vi "Untitled 2.vi"() -> ()   [LabVIEW 2017]
uses:
  <vilib>/myRIO/Common/Instrument Driver Framework/myRIO v1.0/Encoder/typedefs/Encoder Signal Mode.ctl
  <vilib>/myRIO/Instrument Drivers/Onboard IO/Encoder/typedefs/Encoder Reference.ctl
  <vilib>/myRIO/Common/Instrument Driver Framework/Utilities/typedefs/myRIO Generic Hardware Reference.ctl
  <vilib>/myRIO/Common/Instrument Driver Framework/Utilities/typedefs/Hardware Version Enum.ctl
  <vilib>/myRIO/Common/Instrument Driver Framework/Utilities/typedefs/myRIO v1.0 Reference.ctl
  <vilib>/myRIO/Common/Instrument Driver Framework/Utilities/typedefs/Generic FPGA Reference.ctl
  <vilib>/myRIO/Common/Instrument Driver Framework/myRIO v1.0/Encoder/typedefs/Encoder Channels Enum.ctl
  <vilib>/myRIO/Common/Instrument Driver Framework/myRIO v1.0/Encoder/typedefs/Encoder Configuration v1.0.ctl
  <vilib>/userdefined/High Color/nirio_resource_hc.ctl
  <vilib>/myRIO/Common/Instrument Driver Framework/Utilities/vis/Is FPGA Ref Available.vi
  <vilib>/myRIO/Common/Instrument Driver Framework/myRIO v1.0/Encoder/vis/myRIO v1.1 Open Encoder.vi
  <vilib>/myRIO/Instrument Drivers/Onboard IO/Encoder/vis/Read.vi
  <vilib>/myRIO/Common/Instrument Driver Framework/Utilities/vis/Validate Channels.vi
  <vilib>/myRIO/Common/Instrument Driver Framework/myRIO v1.0/Encoder/vis/myRIO v1.0 Reserve Encoder.vi
  <vilib>/myRIO/Common/Instrument Driver Framework/myRIO v1.0/Encoder/vis/myRIO v1.0 Build MUX Configuration Encoder.vi
  <vilib>/myRIO/Common/Instrument Driver Framework/myRIO v1.0/Resource Manager/vis/myRIO v1.0 Reserve Channel List.vi
  <vilib>/myRIO/Common/Instrument Driver Framework/myRIO v1.0/Resource Manager/vis/myRIO v1.0 Create Configuration List.vi
  <vilib>/myRIO/Common/Instrument Driver Framework/myRIO v1.0/Resource Manager/vis/myRIO v1.0 Reserve Channel.vi
  <vilib>/myRIO/Common/Instrument Driver Framework/myRIO v1.0/Resource Manager/vis/myRIO v1.0 Unreserve Channel.vi
  <vilib>/myRIO/Common/Instrument Driver Framework/myRIO v1.0/Resource Manager/vis/myRIO v1.0 Build Mutex Name.vi
  <vilib>/Utility/VariantDataType/GetNumericInfo.vi
  <vilib>/Utility/error.llb/Error Cluster From Error Code.vi
  <vilib>/myRIO/Common/Instrument Driver Framework/myRIO v1.0/myRIO v1.1 Open.vi
  <vilib>/myRIO/Common/Instrument Driver Framework/Utilities/vis/IO Manager.vi
  <vilib>/myRIO/Common/Instrument Driver Framework/Utilities/vis/Configuration Manager.vi
  <vilib>/myRIO/Common/Instrument Driver Framework/myRIO v1.0/Resource Manager/vis/myRIO v1.0 Configure IO.vi
  <vilib>/myRIO/Common/Instrument Driver Framework/myRIO v1.0/myRIO v1.0 Close.vi
  <vilib>/myRIO/Common/Instrument Driver Framework/myRIO v1.0/Encoder/vis/myRIO v1.0 Configure Encoder.vi
  <vilib>/myRIO/Common/Instrument Driver Framework/myRIO v1.0/Encoder/vis/myRIO v1.0 Read Encoder.vi
  <vilib>/addons/control/pid/pid.llb/PID (DBL).vi
  <vilib>/myRIO/Express VI/Onboard IO/Encoder/Encoder Express VI.xnode
  <vilib>/myRIO/Instrument Drivers/Onboard IO/Encoder/vis/myRIO Encoder Open.xnode
  <vilib>/myRIO/Common/Instrument Driver Framework/myRIO v1.0/Encoder/typedefs/Encoder Count Direction Enum.ctl
  <vilib>/addons/control/pid/NI_PID_pid.lvlib
  <vilib>/myRIO/Instrument Drivers/Onboard IO/Encoder/Encoder.lvlib
  <vilib>/Analysis/NI_AALPro.lvlib
  <vilib>/robotics/Navigation/shared/WorldMap/OccupancyGridWorldMap/NI_Robotics_OccupancyGridWorldMap.lvclass
panel:
  out "XY Graph 2":cluster{dbl[], dbl[]}(graph)
  in  "stop 2":bool
  in  "Resolution":dbl=50.0
  out "Intensity Graph":dbl[][](graph)
  out "Frequency":u32=10
  in  "curPos":cluster{"x":i32, "y":i32}
  in  "endPos":cluster{"x":i32, "y":i32}={"x"=0, "y"=6}
  out "path":cluster{"X":i32, "Y":i32}[](array[cluster])
  out "Setpoint B":dbl(slide)=1.3993520911950799 scale=-10.0..10.0
  out "Setpoint A":dbl(slide)=0.6006479088049201 scale=-10.0..10.0
  out "PID B":T1(graph)={"Setpoint"=1.3993520911950799, "output"=0.10115092019020398, "dx/dt"=1.4}
  out "PID A":T1(graph)={"Setpoint"=0.6006479088049201, "output"=0.05446764760463431, "dx/dt"=0.7407999999999447}
  out "OUTPUT A":dbl(slide)=0.7407999999999447 scale=-10.0..10.0
  out "OUTPUT B":dbl(slide)=1.4 scale=-10.0..10.0
  in  "stop":bool
  in  "PID gains":T2={"proportional gain (Kc)"=0.05, "integral time (Ti, min)"=0.05, "derivative time (Td, min)"=0.0} {"derivative time (Td, min)" format="%.3f"; "integral time (Ti, min)" format="%.3f"; "proportional gain (Kc)" format="%.3f"}
  in  "Angle":dbl(slide) scale=-360.0..360.0
  in  "Speed":dbl(slide) scale=-10.0..10.0
  out "X, Y, BEARING 2":cluster{dbl, dbl, dbl}
  out "Final X, Y, BEARING":cluster{dbl, dbl, dbl}
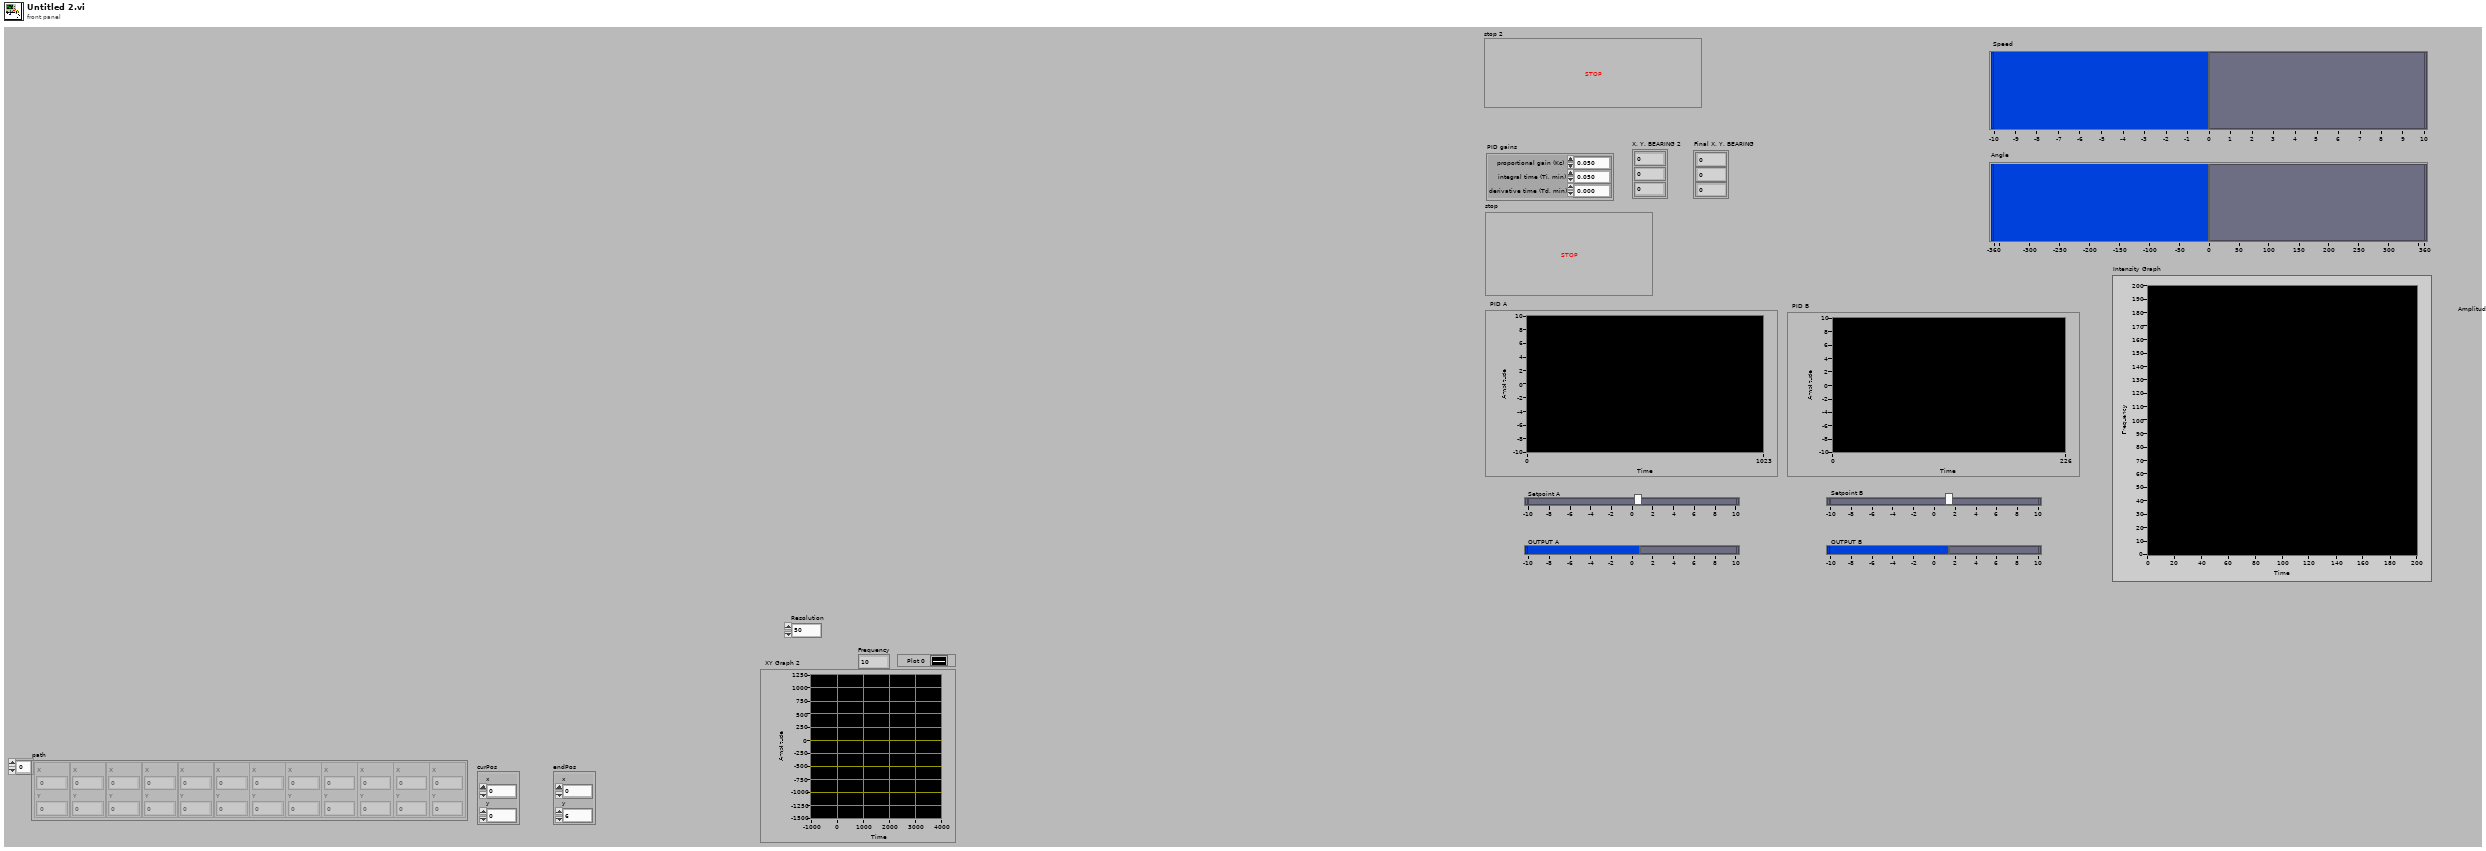
[diagram p1: front panel]
types:
  T1 = cluster{"Setpoint":dbl, "output":dbl, "dx/dt":dbl}
  T2 = cluster{"proportional gain (Kc)":dbl, "integral time (Ti, min)":dbl, "derivative time (Td, min)":dbl}
  T3 = typedef "LidarPoint.ctl" = cluster{"X":dbl, "Y":dbl}
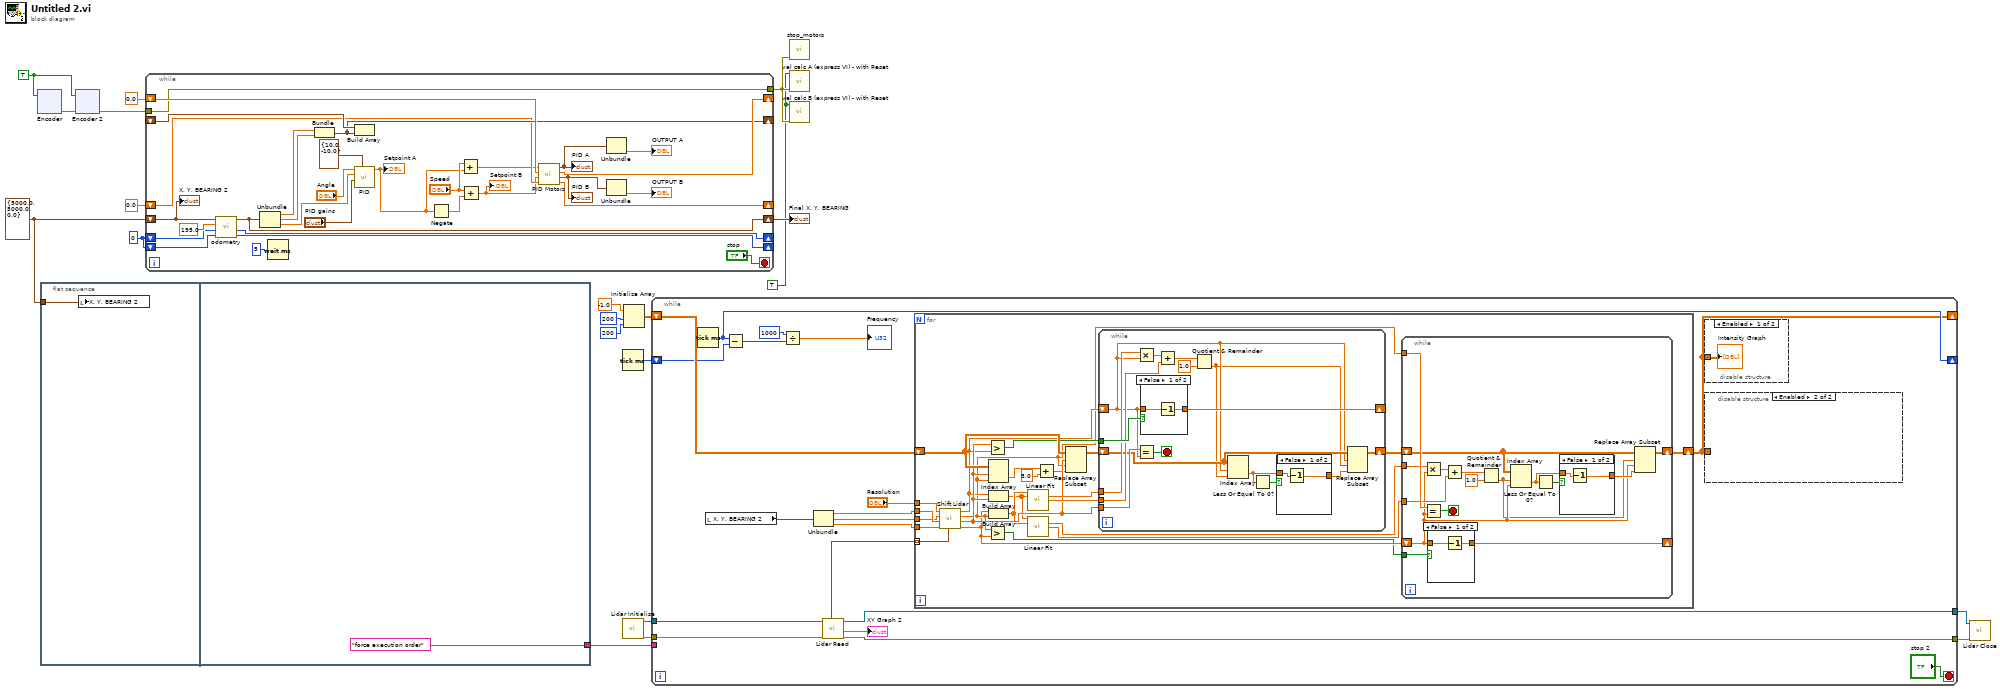
[diagram p0: block diagram]
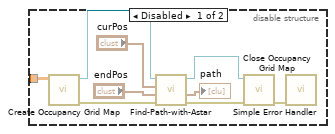
[diagram p2: hidden frame]
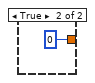
[diagram p4: hidden frame]
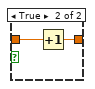
[diagram p5: hidden frame]
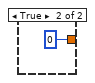
[diagram p6: hidden frame]
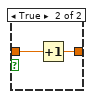
[diagram p7: hidden frame]
diagram:
  w4 = cluster{dbl, dbl, dbl} {5000.0, 5000.0, 0.0} ("Initial X, Y, BEARING")
  w12 = TRUE ("Reinitialise")
  w14 = TRUE
  w16 = 0 ("ENCA OUT")
  n1 = xnode "Encoder"("Reset Counter"=w14) -> ("error out"=w15:errorcluster)  [unwired: 1 in, 3 out]
  n2 = flat-sequence {
    tunnel: w4 -> [w21]
    tunnel: ["force execution order"] -> w3
    frame #0 {
      n3 = local write "X, Y, BEARING 2"(w21) -> ()
    }
    frame #1 {
    }
  }
  n4 = xnode "Encoder 2"("error in (no error)"=w15, "Reset Counter"=w14) -> ("error out"=w13:errorcluster)  [unwired: 3 out]
  n5 = while {
    tunnel: w13 -> [w48]
    shift-right: [w50] -> _
    shift-left: 0.0 ("output A") -> [w51]
    shift-right: [w52] -> _
    shift-left: 0.0 ("output B") -> [w28]
    tunnel: [w48] -> w19
    shift-right: [w40] -> _
    shift-left: w16 -> [w42]
    shift-right: [w39] -> _
    shift-left: w16 -> [w41]
    shift-right: [w38] -> w20
    shift-left: w4 -> [w23]
    shift-right: [w34] -> _
    shift-left: _ -> [w35]
    stop <- "stop" stop-if-true
    n6 = call "odometry.vi"("ENCB in"=w41, "ENCA in"=w42, "wheelbase"=195.0, "Position"=w23) -> ("ENCB OUT"=w39:i32, "ENCA OUT"=w40:i32, "X, Y, BEARING"=w38:cluster{dbl, dbl, dbl})  [unwired: 4 in]
    n7 = Unbundle(w38) -> (w36:dbl, w37:dbl, w32:dbl)
    n8 = Wait (ms)(milliseconds to wait=5 ("ENCB OUT")) -> ()  [unwired: 1 out]
    n9 = Bundle(w36, w37) -> (w34:cluster{dbl, dbl})  [unwired: 1 in]
    n10 = Build Array(w35, w34) -> ()  [unwired: 1 out]
    n11 = call-poly <vilib>:"PID.vi"("output range"=cluster{"output high":dbl, "output low":dbl} {"output high"=10.0, "output low"=-10.0}, "PID gains"="PID gains", "process variable"=w32, "setpoint"="Angle") -> ("output"=w25:dbl)  [unwired: 6 in, 1 out]
    "Setpoint A" <- w25
    n12 = Negate(x=w25) -> (-x=w26:dbl)
    n13 = Add(x="Speed", y=w25) -> (x+y=w24:dbl)
    n14 = Add(x="Speed", y=w26) -> (x+y=w27:dbl)
    "Setpoint B" <- w27
    n15 = call "PID Motors.vi"("input B"=w28, "Speed B"=w27, "input A"=w51, "Speed A"=w24) -> ("output B"=w52:dbl, "Speed B0"=w46:T1, "output A"=w50:dbl, "Speed A0"=w47:T1)
    "PID B" <- w46
    "PID A" <- w47
    n16 = Unbundle(w47) -> ("dx/dt"=→"OUTPUT A":dbl)  [unwired: 2 out]
    n17 = Unbundle(w46) -> ("dx/dt"=→"OUTPUT B":dbl)  [unwired: 2 out]
    "X, Y, BEARING 2" <- w23
  }
  "Final X, Y, BEARING" <- w20
  n18 = Tick Count (ms)() -> (millisecond timer value=w5:u32)
  n19 = call "Lidar Initialise.vi"() -> ("error out"=w10:errorcluster, "VISA resource name out"=w11:refnum<visa-resource-name>)  [unwired: 10 in]
  n20 = Initialize Array(-1.0 ("element"), 200 ("dimension size"), 200 ("dimension size")) -> (w7:dbl[][])
  n21 = while {
    tunnel: w11 -> [w72]
    tunnel: w10 -> [w71]
    shift-right: [w62] -> _
    shift-left: w7 -> [w68]
    shift-right: [w65] -> _
    shift-left: w5 -> [w67]
    tunnel: w3 -> [_]
    tunnel: [w55] -> w2
    tunnel: [w54] -> w1
    stop <- "stop 2" stop-if-true
    n22 = Tick Count (ms)() -> (millisecond timer value=w65:u32)
    n23 = local read "X, Y, BEARING 2"() -> (w59:cluster{dbl, dbl, dbl})
    n24 = Subtract(x=w65, y=w67) -> (x-y=w64:u32)
    n25 = Divide(x=u32 1000 ("y"), y=w64) -> (x/y=→"Frequency":dbl)
    n26 = Unbundle(w59) -> (w58:dbl, w57:dbl, w56:dbl)
    n27 = call "Lidar Read.vi"("error in (no error)"=w71, "VISA resource name"=w72) -> ("error out"=w55:errorcluster, "Visual Out"=→"XY Graph 2":cluster{dbl[], dbl[]}, "VISA resource name out"=w54:refnum<visa-resource-name>, "XYflipped"=w60:T3[])  [unwired: 2 in, 3 out]
    n28 = for {
      tunnel: "Resolution" -> [w106]
      tunnel: w60 -> [w105] mode=indexing
      shift-right: [w93] -> w62
      shift-left: w68 -> [w104]
      tunnel: w58 -> [w85]
      tunnel: w57 -> [w84]
      tunnel: w56 -> [w83]
      n29 = call "Shift Lidar.vi"("XY"=w105, "Angle"=w83, "X position"=w85, "Y position"=w84, "Resolution"=w106) -> ("PosY"=w91:dbl, "Shifted X"=w101:dbl, "Shifted Y"=w92:dbl, "PosX"=w98:dbl)  [unwired: 3 in]
      n30 = Greater?(x=w101, y=w98) -> (0:w100:bool)
      n31 = Greater?(x=w92, y=w91) -> (0:w90:bool)
      n32 = Index Array(array=w104, index (row)=w101, index (col)=w92) -> (element=w97:dbl)
      n33 = Build Array(w98, w101) -> (w88:dbl[])
      n34 = Build Array(w91, w92) -> (w89:dbl[])
      n35 = call <vilib>:"Linear Fit.vi"("Y"=w89, "X"=w88) -> ("slope"=w103:dbl, "intercept"=w102:dbl)  [unwired: 9 in, 3 out]
      n36 = call <vilib>:"Linear Fit.vi"("Y"=w88, "X"=w89) -> ("slope"=w87:dbl, "intercept"=w86:dbl)  [unwired: 9 in, 3 out]
      n37 = Add(x=w97, y=5.0) -> (x+y=w96:dbl)
      n38 = Replace Array Subset(array=w104, new element=w96, index (row)=w101, index (col)=w92) -> (w99:dbl[][])
      n39 = while {
        tunnel: w101 -> [w144]
        shift-right: [w142] -> _
        shift-left: w98 -> [w137]
        tunnel: w103 -> [w141]
        tunnel: w102 -> [w139]
        tunnel: w100 -> [w143]
        shift-right: [w136] -> w94
        shift-left: w99 -> [w138]
        stop <- w145 stop-if-true
        n40 = Multiply(x=w141, y=w137) -> (x*y=w140:dbl)
        n41 = Equal?(x=w144, y=w137) -> (x = y?=w145:bool)
        n42 = case shown="False" w143 {
          tunnel: w137 -> [w149 w152]
          tunnel: [w150 w151] -> w142
          frame False {
            n43 = Decrement(x=w149) -> (x-1=w150:dbl)
          }
          frame True {
            n44 = Increment(x=w152) -> (x+1=w151:dbl)
          }
        }
        n45 = Add(x=w140, y=w139) -> (x+y=w132:dbl)
        n46 = Quotient & Remainder(x=w132, y=1.0) -> (floor(x/y)=w130:dbl)  [unwired: 1 out]
        n47 = Index Array(array=w138, index (row)=w137, index (col)=w130) -> (element=w133:dbl)
        n48 = Less Or Equal To 0?(x=w133) -> (x <= 0?=w135:bool)
        n49 = case shown="False" w135 {
          tunnel: [w147 0] -> w134
          tunnel: w133 -> [w146 _]
          frame False {
            n50 = Decrement(x=w146) -> (x-1=w147:dbl)
          }
          frame True {
          }
        }
        n51 = Replace Array Subset(array=w138, new element=w134, index (row)=w137, index (col)=w130) -> (w136:dbl[][])
      }
      n52 = while {
        shift-right: [w111] -> w93
        shift-left: w94 -> [w110]
        shift-right: [w119] -> _
        shift-left: w91 -> [w108]
        tunnel: w92 -> [w121]
        tunnel: w90 -> [w120]
        tunnel: w87 -> [w118]
        tunnel: w86 -> [w116]
        stop <- w122 stop-if-true
        n53 = Multiply(x=w118, y=w108) -> (x*y=w117:dbl)
        n54 = Equal?(x=w121, y=w108) -> (x = y?=w122:bool)
        n55 = case shown="False" w120 {
          tunnel: w108 -> [w126 w129]
          tunnel: [w127 w128] -> w119
          frame False {
            n56 = Decrement(x=w126) -> (x-1=w127:dbl)
          }
          frame True {
            n57 = Increment(x=w129) -> (x+1=w128:dbl)
          }
        }
        n58 = Add(x=w117, y=w116) -> (x+y=w115:dbl)
        n59 = Quotient & Remainder(x=w115, y=1.0) -> (floor(x/y)=w107:dbl)  [unwired: 1 out]
        n60 = Index Array(array=w110, index (row)=w107, index (col)=w108) -> (element=w112:dbl)
        n61 = Less Or Equal To 0?(x=w112) -> (x <= 0?=w113:bool)
        n62 = case shown="False" w113 {
          tunnel: [w124 0] -> w109
          tunnel: w112 -> [w123 _]
          frame False {
            n63 = Decrement(x=w123) -> (x-1=w124:dbl)
          }
          frame True {
          }
        }
        n64 = Replace Array Subset(array=w110, new element=w109, index (row)=w107, index (col)=w108) -> (w111:dbl[][])
      }
    }
    n65 = disable-structure shown="Enabled" {
      disable-tunnel: w62 -> [w82 _]
      frame Enabled {
        "Intensity Graph" <- w82
      }
      frame Disabled {
      }
    }
    n66 = disable-structure shown="Enabled" {
      disable-tunnel: w62 -> [w73 _]
      frame Disabled {
        n67 = call <vilib>:"Create Occupancy Grid Map.vi"("occupancy grid"=w73) -> ("error out"=w81:errorcluster, "map reference out"=w78:refnum<data-value>)  [unwired: 9 in]
        n68 = call "Find-Path-with-Astar.vi"("error in (no error)"=w81, "goal node"="endPos", "start node"="curPos", "map reference in"=w78) -> ("error out"=w76:errorcluster, "Array"=→"path":cluster{"X":i32, "Y":i32}[], "map reference out"=w77:refnum<data-value>)  [unwired: 5 in]
        n69 = call <vilib>:"Close Occupancy Grid Map.vi"("error in (no error)"=w76, "map reference in"=w77) -> ("error out"=w75:errorcluster)  [unwired: 9 in]
        n70 = call <vilib>:"Simple Error Handler.vi"("error in (no error)"=w75) -> ()  [unwired: 4 in, 5 out]
      }
      frame Enabled {
      }
    }
  }
  n71 = call "stop_motors.vi"("error in (no error)"=w19) -> ()  [unwired: 4 in, 1 out]
  n72 = call "vel calc A (express VI) - with Reset.vi"("error in"=w19, "Reinitialise"=w12) -> ()  [unwired: 5 in, 5 out]
  n73 = call "vel calc B (express VI) - with Reset.vi"("error in"=w19, "Reinitialise"=w12) -> ()  [unwired: 5 in, 5 out]
  n74 = call "Lidar Close.vi"("error in (no error)"=w2, "VISA resource name"=w1) -> ()  [unwired: 9 in, 1 out]
